vi "Read Test Report.vi"(8 "error in (no error)":errorcluster, 11 "Test Runner in":refnum<class "Test Runner.lvclass">) -> (0 "error out":errorcluster, 2 "Test Report":refnum<class "Test Report.lvclass">, 3 "Test Runner out":refnum<class "Test Runner.lvclass">)   [LabVIEW 2013, in "Caraya.lvlib" / "Test Runner.lvclass"]
uses:
  Test Runner.lvclass
  Test Report/Test Report.lvclass
  Test Runner.lvclass/Test Runner.ctl
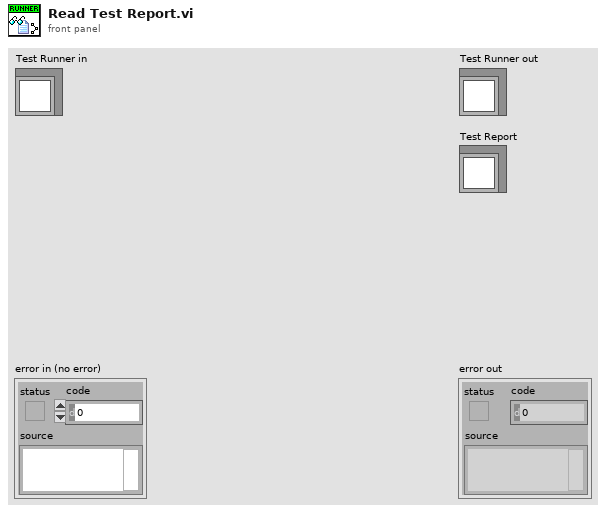
[diagram p1: front panel]
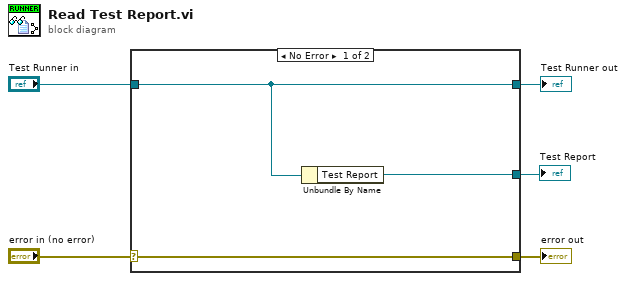
[diagram p0: block diagram]
diagram:
  n1 = case shown="No Error" "error in (no error)" {
    selector: "error in (no error)" -> [w8 w9]
    tunnel: [w8 w9] -> w4
    tunnel: [w7 w10] -> w2
    tunnel: "Test Runner in" -> [w7 w10]
    tunnel: [w6 _] -> w1
    frame No Error {
      n2 = Unbundle By Name(w7) -> ("Test Report"=w6:refnum<class "Test Report.lvclass">)
    }
    frame Error {
    }
  }
  "error out" <- w4
  "Test Runner out" <- w2
  "Test Report" <- w1
